vi "摄氏华氏.vi"() -> ()   [LabVIEW 2020]
panel:
  out "华氏温度":dbl
  in  "摄氏温度":dbl
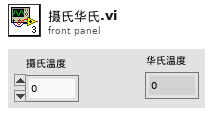
[diagram p1: front panel]
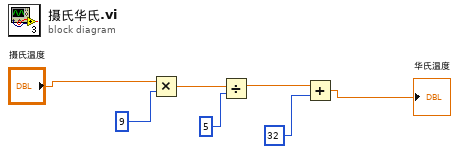
[diagram p0: block diagram]
diagram:
  n1 = Multiply(x="摄氏温度", y=9) -> (x*y=w5:dbl)
  n2 = Divide(x=w5, y=5) -> (x/y=w3:dbl)
  n3 = Add(x=w3, y=32) -> (x+y=→"华氏温度":dbl)
